vi "OnDataChange.vi"(0 "QuickNote in":refnum<class "QuickNote.lvclass">, 1 "DataExchange":T1, 3 "error in (no error)":errorcluster) -> (7 "QuickNote out":refnum<class "QuickNote.lvclass">, 10 "error out":errorcluster)   [LabVIEW 2020, in "QuickNote.lvlib" / "QuickNote.lvclass"]
uses:
  QuickNote.lvclass
  Hardware Abstraction Layer/Component/Device/Device/DataExchange.ctl
  QuickNote.lvclass/QuickNote.ctl
  Hardware Abstraction Layer/Component/GenericActor/GenericActor/GenericActor.lvclass
  Interface/DataListener/DataListener.lvclass
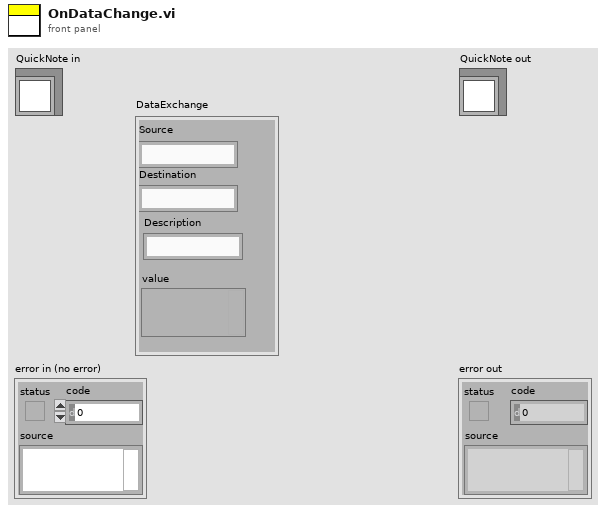
[diagram p1: front panel]
types:
  T1 = typedef "DataListener.lvclass/DataExchange.ctl" = cluster{"Source":string, "Destination":string, "Description":string, "value":variant}
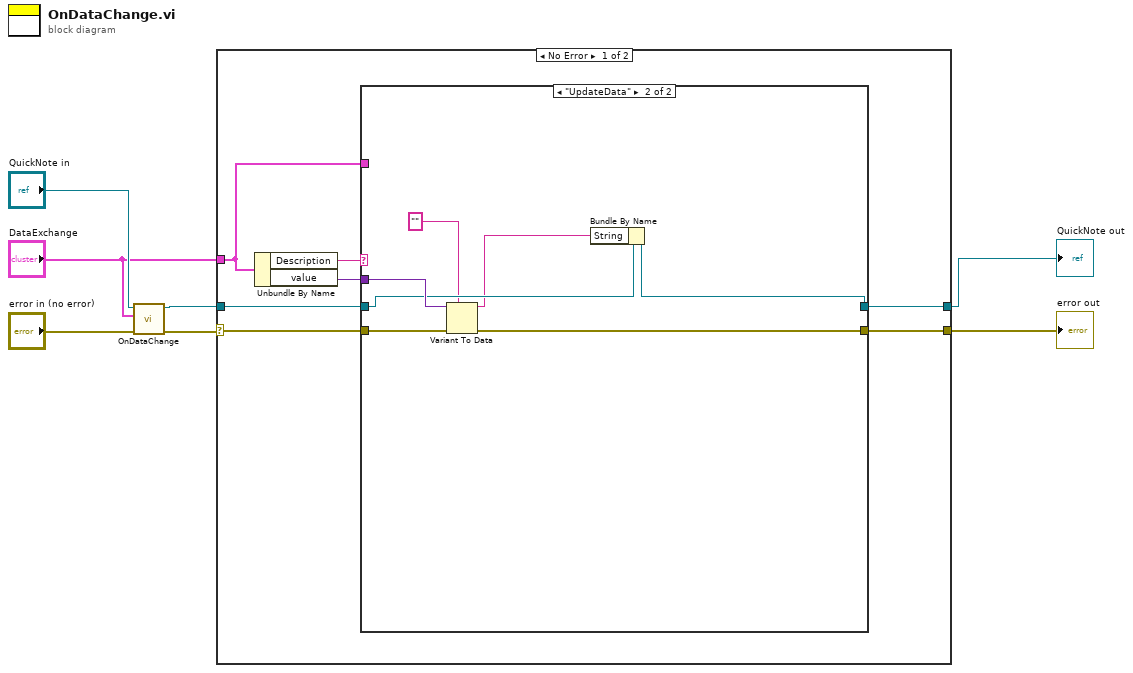
[diagram p0: block diagram]
diagram:
  n1 = call-parent "OnDataChange.vi"("GRMActor in"="QuickNote in", "DataExchange"="DataExchange", "error in (no error)"="error in (no error)") -> ("GRMActor out"=w4:refnum<class "QuickNote.lvclass">, "error out"=w5:errorcluster)  [unwired: 6 in]
  n2 = case shown="No Error" w5 {
    selector: w5 -> [w12 w25]
    tunnel: [w13 w25] -> w2
    tunnel: w4 -> [w9 w24]
    tunnel: [w14 w24] -> w1
    tunnel: "DataExchange" -> [w8 _]
    frame No Error {
      n3 = Unbundle By Name(w8) -> ("Description"=w11:string, "value"=w10:variant)
      n4 = case shown="\"UpdateData\"" w11 {
        tunnel: w10 -> [_ w22]
        tunnel: [w16 w19] -> w14
        tunnel: w9 -> [w16 w20]
        tunnel: [w15 w21] -> w13
        tunnel: w12 -> [w15 w23]
        tunnel: w8 -> [_ _]
        frame Default {
        }
        frame "UpdateData" {
          n5 = Variant To Data(error in=w23, type="" ("String"), Variant=w22) -> (data=w17:string, error out=w21:errorcluster)
          n6 = Bundle By Name(cluster=w20, "String"=w17) -> (w19:refnum<class "QuickNote.lvclass">)
        }
      }
    }
    frame Error {
    }
  }
  "error out" <- w2
  "QuickNote out" <- w1
